vi "STM Read Meta Data (Serial Clst).vi"(6 "Options":T3={"Ignore Timeout Error"=TRUE, "timeout ms (1000)"=1000}, 8 "error in":errorcluster, 11 "Connection Info In":T1) -> (0 "error out":errorcluster, 1 "Meta data":T2[](array[typedef]), 3 "Connection Info Out":T1)   [LabVIEW 2014, in "QwaveSys Raspberry Pi Library.lvlib"]
doc: "This VI reads the meta data information from a remote computer. Use this VI to retrieve the variable names and types that a remote computer exports.\n\nThis VI parses the data and returns a cluster containing the meta data information."
uses:
  QwaveSys Raspberry Pi Library.lvlib
  _SubVIs/stm_MetaDataElement.ctl
  stm_Serial Read Options.ctl
  stm_Serial Connection Info.ctl
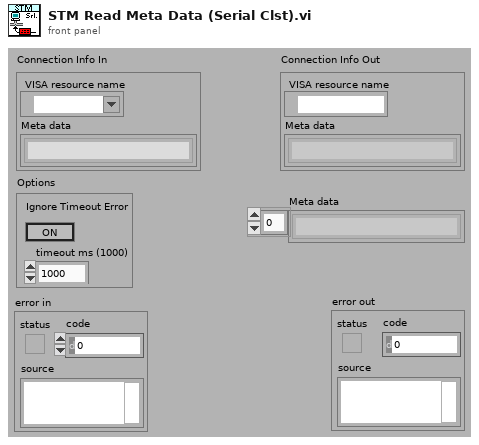
[diagram p1: front panel]
types:
  T1 = typedef "QwaveSys Raspberry Pi Library.lvlib/stm_Serial Connection Info.ctl" = cluster{"VISA resource name":refnum<visa-resource-name>, "Meta data":T2[]}
  T2 = typedef "QwaveSys Raspberry Pi Library.lvlib/stm_MetaDataElement.ctl" = string
  T3 = typedef "QwaveSys Raspberry Pi Library.lvlib/stm_Serial Read Options.ctl" = cluster{"Ignore Timeout Error":bool, "timeout ms (1000)":u32}
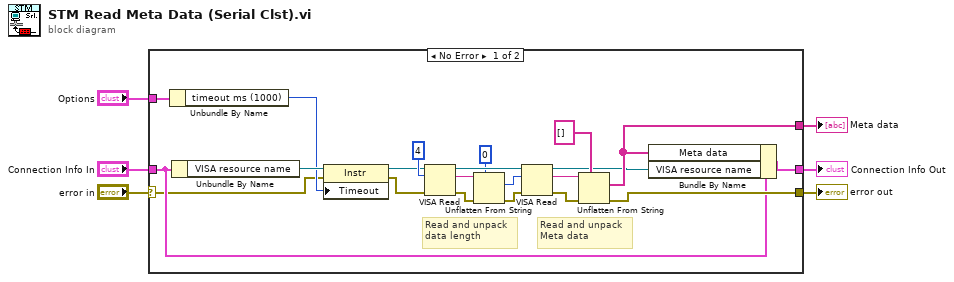
[diagram p0: block diagram]
diagram:
  n1 = case shown="No Error" "error in" {
    selector: "error in" -> [w8 w29]
    tunnel: [w16 _] -> w6
    tunnel: [w27 w29] -> w5
    tunnel: [w14 w28] -> w1
    tunnel: "Options" -> [w13 _]
    tunnel: "Connection Info In" -> [w12 w28]
    frame No Error {
      # "Read and unpack\nMeta data"
      # "Read and unpack\ndata length"
      n2 = Unbundle By Name(w13) -> ("timeout ms (1000)"=w9:u32)
      n3 = Unbundle By Name(w12) -> ("VISA resource name"=w11:refnum<visa-resource-name>)
      n4 = property class="Instr"(reference=w11, error in=w8, "Timeout"=w9) -> (reference out=w10:refnum<visa-resource-name>, error out=w7:errorcluster)
      n5 = VISA Read(VISA resource name=w10, byte count=u32 4 ("bytes to read"), error in (no error)=w7) -> (VISA resource name out=w24:refnum<visa-resource-name>, read buffer=w21:string, error out=w17:errorcluster)  [unwired: 1 out]
      n6 = Unflatten From String(type=u32 0 ("bytes to read"), binary string=w21, error in (no error)=w17) -> (value=w18:u32, error out=w19:errorcluster)  [unwired: 3 out]
      n7 = VISA Read(VISA resource name=w24, byte count=w18, error in (no error)=w19) -> (VISA resource name out=w15:refnum<visa-resource-name>, read buffer=w23:string, error out=w22:errorcluster)  [unwired: 1 out]
      n8 = Unflatten From String(type=T2[] [] ("Meta data"), binary string=w23, error in (no error)=w22) -> (value=w16:T2[], error out=w27:errorcluster)  [unwired: 3 out]
      n9 = Bundle By Name(cluster=w12, "Meta data"=w16, "VISA resource name"=w15) -> (w14:T1)
    }
    frame Error {
    }
  }
  "Meta data" <- w6
  "error out" <- w5
  "Connection Info Out" <- w1
